vi "SaveModificationConditionFonctionnelle.vi"(8 "error In":errorcluster, 10 "Ident cond.Fonctionnelle":T5, 11 "Condition fonctionnelle":T1) -> (0 "error Out":errorcluster)   [LabVIEW 2009]
uses:
  Param_PopupEditLimitesConditionFonctionnelle.ctl
  LIBRAIRIE/010_DATABASE/30_ABAQUES/DB_Abaque_ConditionFonctionnelle.ctl
  LIBRAIRIE/010_DATABASE/50_STATISTIQUES/020_STATISTIQUES/Ctrl/STAT_ConditionFonctionnelle.ctl
  LIBRAIRIE/010_DATABASE/50_STATISTIQUES/020_STATISTIQUES/Ctrl/STAT_Limite.ctl
  LIBRAIRIE/010_DATABASE/50_STATISTIQUES/020_STATISTIQUES/Ctrl/STAT_Enum_Criticité.ctl
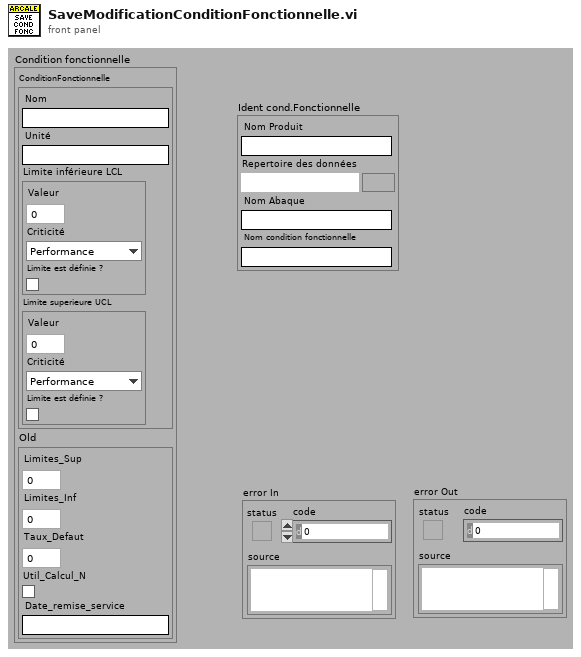
[diagram p1: front panel]
types:
  T1 = typedef "DB_Abaque_ConditionFonctionnelle.ctl" = cluster{"ConditionFonctionnelle":T2, "Old":cluster{"Limites_Sup":dbl, "Limites_Inf":dbl, "Taux_Defaut":dbl, "Util_Calcul_N":bool, "Date_remise_service":string}}
  T2 = typedef "STAT_ConditionFonctionnelle.ctl" = cluster{"Nom":string, "Unité":string, "Limite inférieure LCL":T3, "Limite superieure UCL":T3}
  T3 = typedef "STAT_Limite.ctl" = cluster{"Valeur":dbl, "Criticité":T4, "Limite est définie ?":bool}
  T4 = typedef "STAT_Enum_Criticité.ctl" = enum16{"Performance", "Working", "Safety"}
  T5 = typedef "Param_PopupEditLimitesConditionFonctionnelle.ctl" = cluster{"Nom Produit":string, "Repertoire des données":path, "Nom Abaque":string, "Nom condition fonctionnelle":string}
  T6 = typedef "DB_Abaque.ctl" = cluster{"Nom":string, "TabCalculs":T7[]}
  T7 = typedef "DB_Abaque_Calcul.ctl" = cluster{"Index":string, "Nom":string, "Expression":string, "Condition fonctionnelle existe ?":bool, "Condition fonctionnelle":T1}
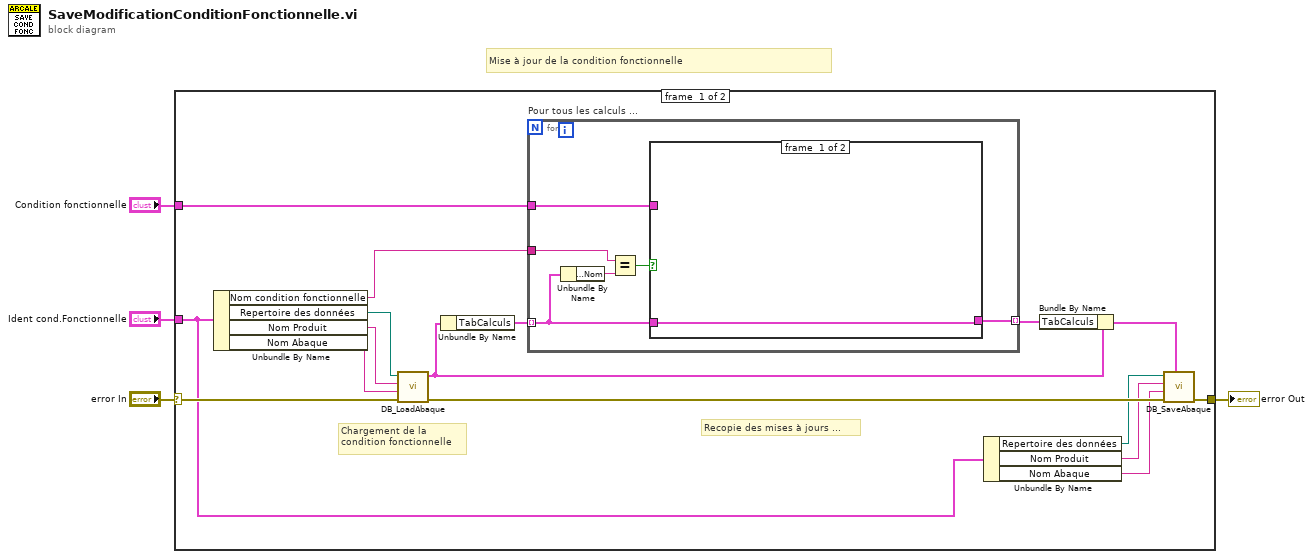
[diagram p0: block diagram]
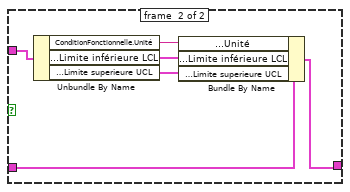
[diagram p2: hidden frame]
diagram:
  # "Mise à jour de la condition fonctionnelle"
  n1 = case shown="No Error" "error In" {
    selector: "error In" -> [w20 w34]
    tunnel: [w10 w34] -> w3
    tunnel: "Ident cond.Fonctionnelle" -> [w8 _]
    tunnel: "Condition fonctionnelle" -> [w15 _]
    frame #0 {
      # "Recopie des mises à jours ..."
      # "Chargement de la\ncondition fonctionnelle"
      n2 = Unbundle By Name(w8) -> ("Nom condition fonctionnelle"=w14:string, "Repertoire des données"=w19:path, "Nom Produit"=w18:string, "Nom Abaque"=w17:string)
      n3 = call "DB_LoadAbaque.vi"("error in (no error)"=w20, "Nom Abaque"=w17, "Nom Produit"=w18, "Repertoire des données"=w19) -> ("error out"=w11:errorcluster, "Abaque"=w12:T6)  [unwired: 6 in]
      n4 = Unbundle By Name(w12) -> ("TabCalculs"=w16:T7[])
      n5 = for "Pour tous les calculs ..." {
        tunnel: w16 -> [w22] mode=indexing
        tunnel: w15 -> [w23]
        tunnel: w14 -> [w25]
        tunnel: [w21] -> w13 mode=indexing
        n6 = Unbundle By Name(w22) -> ("Condition fonctionnelle.ConditionFonctionnelle.Nom"=w26:string)
        n7 = Equal?(x=w25, y=w26) -> (x = y?=w24:bool)
        n8 = case shown="True" w24 {
          tunnel: w23 -> [_ w33]
          tunnel: w22 -> [w27 w32]
          tunnel: [w27 w28] -> w21
          frame #0 {
          }
          frame #1 {
            n9 = Unbundle By Name(w33) -> ("ConditionFonctionnelle.Unité"=w31:string, "ConditionFonctionnelle.Limite inférieure LCL"=w30:T3, "ConditionFonctionnelle.Limite superieure UCL"=w29:T3)
            n10 = Bundle By Name(cluster=w32, "Condition fonctionnelle.ConditionFonctionnelle.Unité"=w31, "Condition fonctionnelle.ConditionFonctionnelle.Limite inférieure LCL"=w30, "Condition fonctionnelle.ConditionFonctionnelle.Limite superieure UCL"=w29) -> (w28:T7)
          }
        }
      }
      n11 = Unbundle By Name(w8) -> ("Repertoire des données"=w7:path, "Nom Produit"=w6:string, "Nom Abaque"=w5:string)
      n12 = Bundle By Name(cluster=w12, "TabCalculs"=w13) -> (w9:T6)
      n13 = call "DB_SaveAbaque.vi"("Abaque"=w9, "error in (no error)"=w11, "Nom Abaque"=w5, "Nom Produit"=w6, "Repertoire des données"=w7) -> ("error out"=w10:errorcluster)  [unwired: 6 in]
    }
    frame #1 {
    }
  }
  "error Out" <- w3
